vi "Remove Range.vi"(8 "error in (no error)":errorcluster caption="错误输入（无错误）", 10 "Keys":string[](array[string]), 11 "Dictionary In":refnum<class "Dictionary.lvclass"> caption="DNL_LabVIEW Object in") -> (0 "error out":errorcluster caption="错误输出", 1 "Key Exist?":bool, 2 "Removed Values":string[](array[string]), 3 "Dictionary Out":refnum<class "Dictionary.lvclass"> caption="DNL_LabVIEW Object out")   [LabVIEW 2012, in "Dictionary.lvclass"]
uses:
  Dictionary.lvclass
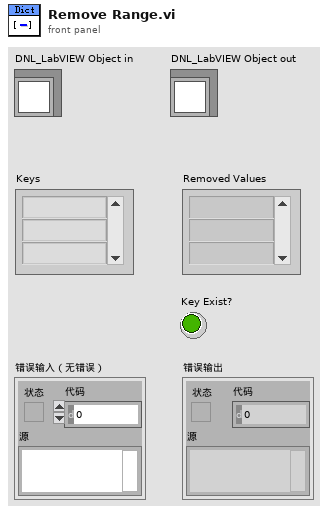
[diagram p1: front panel]
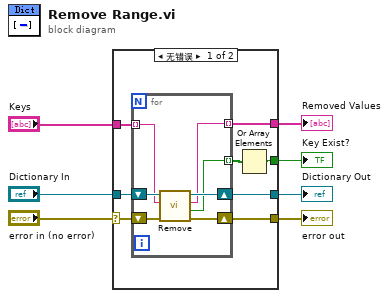
[diagram p0: block diagram]
diagram:
  n1 = case shown="无错误" "error in (no error)" {
    selector: "error in (no error)" -> [w13 w24]
    tunnel: [w12 w24] -> w6
    tunnel: [w11 w23] -> w4
    tunnel: "Dictionary In" -> [w14 w23]
    tunnel: "Keys" -> [w15 _]
    tunnel: [w10 _] -> w2
    tunnel: [w8 _] -> w1
    frame No Error {
      n2 = for {
        tunnel: w15 -> [w18] mode=indexing
        shift-right: [w21] -> w11
        shift-left: w14 -> [w22]
        shift-right: [w19] -> w12
        shift-left: w13 -> [w20]
        tunnel: [w17] -> w10 mode=indexing
        tunnel: [w16] -> w9 mode=indexing
        n3 = call "Remove.vi"("error in (no error)"=w20, "Key"=w18, "Dictionary In"=w22) -> ("error out"=w19:errorcluster, "Key Exist?"=w16:bool, "Removed Value"=w17:string, "Dictionary Out"=w21:refnum<class "Dictionary.lvclass">)  [unwired: 5 in]
      }
      n4 = Or Array Elements(Boolean array=w9) -> (logical OR=w8:bool)
    }
    frame Error {
    }
  }
  "error out" <- w6
  "Dictionary Out" <- w4
  "Key Exist?" <- w1
  "Removed Values" <- w2
